vi "Begin.vi"() -> (0 "error out":errorcluster)   [LabVIEW 2012]
doc: "Called before other user functions, this VI is expected to open initial I/O refnums, load in file data, and do all program initialization. Notice that the <B>error out</B> terminal is simply used for data flow. Wiring it to other structures or subVIs ensures that this VI runs first."
uses:
  <vilib>/Rock Robotics/WPI/DriverStation/WPI_DriverStationRobotMode2.ctl
  <vilib>/Rock Robotics/WPI/Joystick/WPI_JoystickDeviceEnum.ctl
  <vilib>/Rock Robotics/SystemInterfaces/DIO/FPGA_DIOPWMChannel.ctl
  <vilib>/Rock Robotics/SystemInterfaces/DIO/FPGA_DIORelayChannel.ctl
  <vilib>/Rock Robotics/WPI/Relay/WPI_RelayDirection.ctl
  <vilib>/Rock Robotics/SystemInterfaces/DIO/FPGA_DIOChannel.ctl
  <vilib>/Rock Robotics/WPI/Encoder/WPI_EncoderType.ctl
  <vilib>/Rock Robotics/SystemInterfaces/AI/FPGA_AIGyroChannel.ctl
  <vilib>/Rock Robotics/WPI/Solenoid/WPI_SolenoidChannel.ctl
  <vilib>/Rock Robotics/SystemInterfaces/Typedef/FPGA_TypedefSolenoidModule.ctl
  Robot Global Data.vi
  <vilib>/Rock Robotics/WPI/RobotDrive/WPI_RobotDriveOpen4MotorWithTalon.vi
  <vilib>/Rock Robotics/WPI/Solenoid/WPI_SolenoidOpenSingle.vi
  <vilib>/Rock Robotics/WPI/Solenoid/Deprecated/WPI_SolenoidSetBool.vi
  <vilib>/Rock Robotics/WPI/Counter/WPI_CounterDigitalInputToDigitalSource.vi
  <vilib>/Rock Robotics/WPI/MotorControl/WPI_MotorControlOpen Jaguar.vi
  <vilib>/Rock Robotics/WPI/Compressor/WPI_CompressorGetSetRefNum.vi
  <vilib>/Rock Robotics/SystemInterfaces/Typedef/FPGA_TypedefDigitalModule.ctl
  <vilib>/Rock Robotics/WPI/MotorControl/WPI_MotorControlOpen Talon.vi
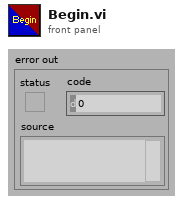
[diagram p1: front panel]
types:
  T1 = cluster{"Target Voltage":dbl, "Target Speed":dbl, "Angle Up?":bool}
  T2 = typedef "FPGA_DIOChannel.ctl" = enum8{"DIO 1", "DIO 2", "DIO 3", "DIO 4", "DIO 5", "DIO 6", "DIO 7", "DIO 8", "DIO 9", "DIO 10", "DIO 11", "DIO 12", "DIO 13", "DIO 14", "Invalid"}
  T3 = typedef "WPI_SolenoidChannel.ctl" = enum8{"Solenoid 1", "Solenoid 2", "Solenoid 3", "Solenoid 4", "Solenoid 5", "Solenoid 6", "Solenoid 7", "Solenoid 8", "Invalid"}
  T4 = typedef "FPGA_TypedefSolenoidModule.ctl" = enum16{"Solenoid Module 1", "Solenoid Module 2"}
  T5 = typedef "FPGA_AIGyroChannel.ctl" = enum8{"AI 1", "AI 2", "Invalid"}
  T6 = typedef "WPI_EncoderType.ctl" = enum16{"1x", "2x", "4x"}
  T7 = typedef "FPGA_DIORelayChannel.ctl" = enum8{"Relay 1", "Relay 2", "Relay 3", "Relay 4", "Relay 5", "Relay 6", "Relay 7", "Relay 8", "Invalid"}
  T8 = typedef "WPI_JoystickDeviceEnum.ctl" = enum16{"USB 1", "USB 2", "USB 3", "USB 4", "Kinect 1", "Kinect 2"}
  T9 = typedef "FPGA_DIOPWMChannel.ctl" = enum8{"PWM 1", "PWM 2", "PWM 3", "PWM 4", "PWM 5", "PWM 6", "PWM 7", "PWM 8", "PWM 9", "PWM 10", "Invalid"}
  T10 = typedef "WPI_RelayDirection.ctl" = enum16{"Both directions", "Forward only", "Reverse only"}
  T11 = typedef "WPI_DriverStationRobotMode2.ctl" = enum16{"Autonomous Disabled", "Autonomous Enabled", "Teleop Disabled", "Teleop Enabled", "Timeout", "Finish", "Test Disabled", "Test Enabled"}
  T12 = typedef "WPI_MotorControlDeviceRef.ctl" = cluster{"DeviceStatus":errorcluster, "Type":enum16{"PWM", "CAN"}, "PWM":cluster{"Digital Module":T13, "PWM Channel":T9, "DeadBand":T14}, "CAN":cluster{"Device Number":u8, "Control Mode":T15, "Semaphore":T16, "Max Vout":dbl}, "Invert":bool, "TransformRef":T17, "InvTransformRef":T17}
  T13 = typedef "FPGA_TypedefDigitalModule.ctl" = enum16{"Digital Module 1", "Digital Module 2"}
  T14 = typedef "WPI_PWMDeadband.ctl" = cluster{"Name":string, "maxPositivePwm":i32, "minPositivePwm":i32, "centerPwm":i32, "maxNegativePwm":i32, "minNegativePwm":i32, "angularRange":u16}
  T15 = typedef "WPI_CANJaguar_ControlMode.ctl" = enum8{"Percent VBus", "Current", "Speed", "Position", "Voltage"}
  T16 = typedef "Semaphore RefNum" = refnum<k1>
  T17 = typedef "WPI_PWMTransform_ConPane.ctl" = refnum<vi>
  T18 = typedef "WPI_DigitalInputDevRef.ctl" = cluster{"DevStatus":errorcluster, "DIO Channel":T2, "Digital Module":T13}
  T19 = typedef "WPI_ServoDeviceRef.ctl" = cluster{"DeviceStatus":errorcluster, "Digital Module":T13, "PWM Channel":T9, "DeadBand":T14}
  T20 = typedef "WPI_CompressorDevRef.ctl" = cluster{"DevStatus":errorcluster, "DigitalInputDevRef":T18, "RelayDevRef":T21}
  T21 = typedef "WPI_RelayDevRef.ctl" = cluster{"DevStatus":errorcluster, "Relay Channel":T7, "Digital Module":T13, "Relay Direction":T10}
  T22 = typedef "WPI_JoystickDevRef.ctl" = cluster{"Device":T8}
  T23 = typedef "WPI_SolenoidDevRef.ctl" = cluster{"DevStatus":errorcluster, "Solenoid Module":T4, "Forward Solenoid Channel":T3, "Reverse Solenoid Channel":T3}
  T24 = typedef "FPGA_CounterEncoderSourceConvertionLVSourceType.ctl" = cluster{"DevStatus":errorcluster, "AnalogTriggerMode?":bool, "DigitalMode":cluster{"Digital Module":T13, "DIO Channel":T25}, "AnalogTriggerMode":cluster{"AnalogTriggerIndex":T26, "OutputType":T27}}
  T25 = typedef "FPGA_DIODigitalSourceChannel.ctl" = enum8{"DIO 1", "DIO 2", "DIO 3", "DIO 4", "DIO 5", "DIO 6", "DIO 7", "DIO 8", "DIO 9", "DIO 10", "DIO 11", "DIO 12", "DIO 13", "DIO 14", "Disabled"}
  T26 = typedef "FPGA_AnalogTriggerIndex.ctl" = enum8{"Trig 0", "Trig 1", "Trig 2", "Trig 3", "Trig 4", "Trig 5", "Trig 6", "Trig 7", "Invalid"}
  T27 = typedef "FPGA_AnalogTriggerOutType.ctl" = enum16{"InWindow", "TriggerState", "Rising", "Falling"}
  T28 = typedef "WPI_GyroDevRef.ctl" = cluster{"DevStatus":errorcluster, "Analog Module":T29, "Analog Channel":T30, "Offset":dbl, "Gain (VoltsPerDegree/Second)":dbl}
  T29 = typedef "FPGA_TypedefAnalogModule.ctl" = enum16{"Analog Module 1", "Analog Module 2"}
  T30 = typedef "FPGA_AIChannel.ctl" = enum8{"AI 1", "AI 2", "AI 3", "AI 4", "AI 5", "AI 6", "AI 7", "AI 8", "Invalid"}
  T31 = typedef "WPI_RobotDriveDevRef.ctl" = cluster{"DevStatus":errorcluster, "Motors[]":T12[], "Square Inputs":bool, "Max Output":dbl, "Isochronous":bool}
  T32 = typedef "WPI_EncoderDevRef.ctl" = cluster{"DevStatus":errorcluster, "EncoderIndex":T33, "CounterIndex":T34, "DistancePerCount":dbl, "Decoding Type":T6}
  T33 = typedef "FPGA_EncoderIdx.ctl" = enum8{"Enc 0", "Enc 1", "Enc 2", "Enc 3", "Invalid"}
  T34 = typedef "FPGA_CounterCtrSystemIndex.ctl" = enum8{"Ctr 0", "Ctr 1", "Ctr 2", "Ctr 3", "Ctr 4", "Ctr 5", "Ctr 6", "Ctr 7", "Invalid"}
  T35 = cluster{"Target Voltage":dbl, "Target Speed":i32, "Angle Up?":bool}
  T36 = cluster{"Target Voltage":i32, "Target Speed":i32, "Angle Up?":bool}
  T37 = cluster{"Target Voltage":dbl, "Target Speed":dbl, "Angle Up?":bool}[]
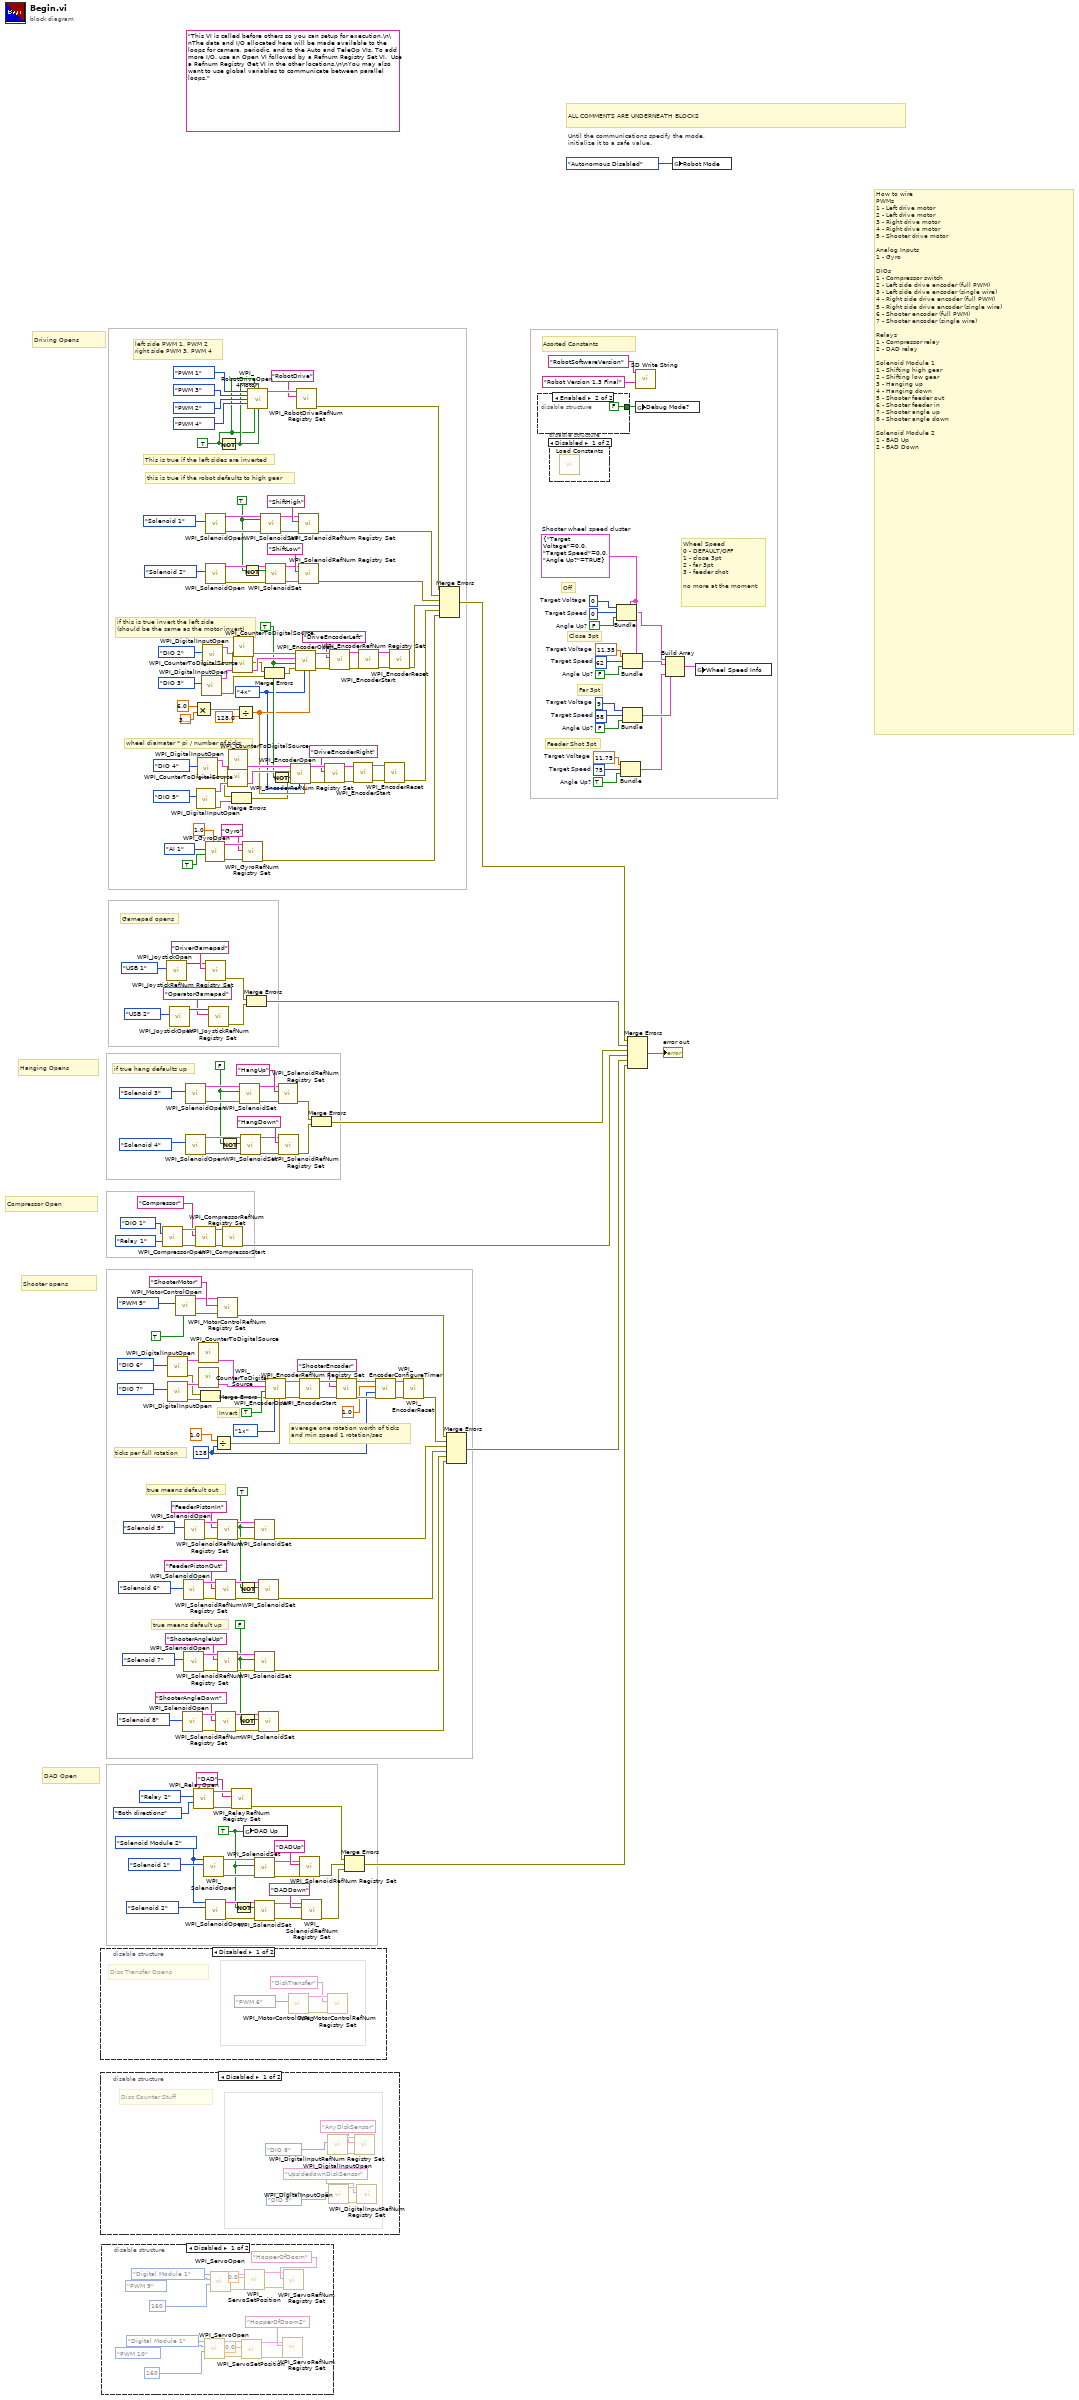
[diagram p0: block diagram]
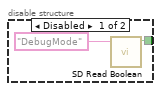
[diagram p2: hidden frame]
diagram:
  w5 = FALSE  # Angle Up?
  w4 = 0  # Target Speed
  w3 = 0  # Target Voltage
  w7 = u8 128 ("Number Samples to Average")
  w14 = TRUE  # Angle Up?
  w15 = 75  # Target Speed
  w16 = 11.75  # Target Voltage
  w19 = FALSE  # Angle Up?
  w18 = 58  # Target Speed
  w17 = 9  # Target Voltage
  w20 = FALSE  # Angle Up?
  w21 = 62  # Target Speed
  w22 = 11.35  # Target Voltage
  w2 = T1 {"Target Voltage"=0.0, "Target Speed"=0.0, "Angle Up?"=TRUE}  # Shooter wheel speed cluster
  w84 = FALSE
  w98 = TRUE
  w57 = TRUE
  w59 = FPGA_TypedefSolenoidModule."Solenoid Module 2" ("Solenoid Module (Module 1)")
  w60 = FALSE
  w62 = WPI_EncoderType."4x" ("Decoding Type")
  w64 = TRUE ("Invert Direction (False)")
  w82 = TRUE
  w80 = TRUE ("Rear Left Motor Inverted")
  (unwired) "This VI is called before others so you can setup for execution.\n\nThe data and I/O allocated here will be made available to the loops for camera, periodic, and to the Auto and TeleOp VIs. To add more I/O, use an Open VI followed by a Refnum Registry Set VI.  Use a Refnum Registry Get VI in the other locations.\n\nYou may also want to use global variables to communicate between parallel loops."
  # "Off"
  # "average one rotation worth of ticks\nand min speed 1 rotation/sec"
  # "Feeder Shot 3pt"
  # "Far 3pt"
  # "Close 3pt"
  # "How to wire\nPWMs\n1 - Left drive motor\n2 - Left drive motor\n3 - Right drive motor\n4 - Right drive motor\n5 - Shooter drive motor\n\nAnalog Inputs\n1 - Gyro\n\nDIOs\n1 - Compressor switch\n2 - Left side drive encoder (full PWM)\n3 - Left side drive encoder (single wire)\n4 - Right side drive encoder (full PWM)\n5 - Right side drive encoder (single wire)\n6 - Shooter encoder (full PWM)\n7 - Shooter encoder (single wire)\n\nRelays\n1 - Compressor relay\n2 - DAD relay\n\nSolenoid Module 1\n1 - Shifting high gear\n2 - Shifting low gear\n3 - Hanging up\n4 - Hanging down\n5 - Shooter feeder out\n6 - Shooter feeder in\n7 - Shooter angle up\n8 - Shooter angle down\n\nSolenoid Module 2\n1 - BAD Up\n2 - BAD Down"
  # "Asorted Constants"
  # "true means default up"
  # "true means default out"
  # "if true hang defaults up"
  # "Gamepad opens"
  # "wheel diamater * pi / number of ticks"
  # "if this is true invert the left side\n(should be the same as the motor invert)"
  # "this is true if the robot defaults to high gear"
  # "left side PWM 1, PWM 2\nright side PWM 3, PWM 4"
  # "This is true if the left sides are inverted"
  # "Compressor Open"
  # "Wheel Speed\n0 - DEFAULT/OFF\n1 - close 3pt\n2 - far 3pt\n3 - feeder shot\n\nno more at the moment"
  # "DAD Open"
  # "Hanging Opens"
  # "Driving Opens"
  # "Shooter opens"
  # "Invert"
  # "ticks per full rotation"
  # "ALL COMMENTS ARE UNDERNEATH BLOCKS"
  # "Until the communications specify the mode,\ninitialize it to a safe value."
  n1 = disable-structure shown="Disabled" {
    frame Disabled {
      # "Disc Transfer Opens"
      n2 = call-poly <vilib>:"WPI_MotorControlOpen.vi"("PWM Channel"=FPGA_DIOPWMChannel."PWM 6") -> ("error out"=w222:errorcluster, "MotorControlDeviceRef"=w223:T12)  [unwired: 9 in]
      n3 = call <vilib>:"WPI_MotorControlRefNum Registry Set.vi"("error in (no error)"=w222, "refnum name"="DiskTransfer", "MotorControlDevRef"=w223) -> ()  [unwired: 7 in, 2 out]
    }
    frame Enabled {
    }
  }
  n4 = disable-structure shown="Disabled" {
    frame Disabled {
      # "Disc Counter Stuff"
      n5 = call <vilib>:"WPI_DigitalInputOpen.vi"("DIO Channel"=FPGA_DIOChannel."DIO 8") -> ("error out"=w232:errorcluster, "DigitalInputDevRef"=w231:T18)  [unwired: 9 in]
      n6 = call <vilib>:"WPI_DigitalInputOpen.vi"("DIO Channel"=FPGA_DIOChannel."DIO 9") -> ("error out"=w230:errorcluster, "DigitalInputDevRef"=w229:T18)  [unwired: 9 in]
      n7 = call <vilib>:"WPI_DigitalInputRefNum Registry Set.vi"("error in (no error)"=w232, "refnum name"="AnyDiskSensor", "DigitalInputDevRef"=w231) -> ()  [unwired: 7 in, 2 out]
      n8 = call <vilib>:"WPI_DigitalInputRefNum Registry Set.vi"("error in (no error)"=w230, "refnum name"="UpsidedownDiskSensor", "DigitalInputDevRef"=w229) -> ()  [unwired: 7 in, 2 out]
    }
    frame Enabled {
    }
  }
  n9 = disable-structure shown="Disabled" {
    frame Disabled {
      n10 = call <vilib>:"WPI_ServoOpen.vi"("Angular Range"=160, "PWM Channel"=FPGA_DIOPWMChannel."PWM 10", "Digital Module (Module 1)"=FPGA_TypedefDigitalModule."Digital Module 1") -> ("error out"=w238:errorcluster, "ServoDeviceRef"=w237:T19)  [unwired: 7 in]
      n11 = call <vilib>:"WPI_ServoOpen.vi"("Angular Range"=160, "PWM Channel"=FPGA_DIOPWMChannel."PWM 9", "Digital Module (Module 1)"=FPGA_TypedefDigitalModule."Digital Module 1") -> ("error out"=w242:errorcluster, "ServoDeviceRef"=w241:T19)  [unwired: 7 in]
      n12 = call <vilib>:"WPI_ServoSetPosition.vi"("error in (no error)"=w238, "Position"=0.0, "ServoDeviceRef"=w237) -> ("error out"=w235:errorcluster, "ServoDeviceRef"=w236:T19)  [unwired: 7 in]
      n13 = call <vilib>:"WPI_ServoSetPosition.vi"("error in (no error)"=w242, "Position"=0.0, "ServoDeviceRef"=w241) -> ("error out"=w240:errorcluster, "ServoDeviceRef"=w239:T19)  [unwired: 7 in]
      n14 = call <vilib>:"WPI_ServoRefNum Registry Set.vi"("error in (no error)"=w235, "refnum name"="HopperOfDoom2", "ServoDeviceRef"=w236) -> ()  [unwired: 7 in, 2 out]
      n15 = call <vilib>:"WPI_ServoRefNum Registry Set.vi"("error in (no error)"=w240, "refnum name"="HopperOfDoom", "ServoDeviceRef"=w239) -> ()  [unwired: 7 in, 2 out]
    }
    frame Enabled {
    }
  }
  n16 = call <vilib>:"WPI_CompressorOpen.vi"("Pressure Switch DIO Channel"=FPGA_DIOChannel."DIO 1", "Relay Channel"=FPGA_DIORelayChannel."Relay 1") -> ("CompressorDevRef"=w164:T20, "error out"=w162:errorcluster)  [unwired: 12 in]
  n17 = call <vilib>:"WPI_JoystickOpen.vi"("JoystickDevice"=WPI_JoystickDeviceEnum."USB 1") -> ("JoystickDevRef"=w218:T22)  [unwired: 10 in]
  n18 = call <vilib>:"WPI_DigitalInputOpen.vi"("DIO Channel"=FPGA_DIOChannel."DIO 6") -> ("error out"=w180:errorcluster, "DigitalInputDevRef"=w193:T18)  [unwired: 9 in]
  n19 = call <vilib>:"WPI_DigitalInputOpen.vi"("DIO Channel"=FPGA_DIOChannel."DIO 7") -> ("error out"=w179:errorcluster, "DigitalInputDevRef"=w189:T18)  [unwired: 9 in]
  n20 = call <vilib>:"WPI_JoystickOpen.vi"("JoystickDevice"=WPI_JoystickDeviceEnum."USB 2") -> ("JoystickDevRef"=w166:T22)  [unwired: 10 in]
  n21 = call-poly <vilib>:"WPI_MotorControlOpen.vi"("Invert"=TRUE, "PWM Channel"=FPGA_DIOPWMChannel."PWM 5") -> ("error out"=w173:errorcluster, "MotorControlDeviceRef"=w174:T12)  [unwired: 8 in]
  n22 = call-poly <vilib>:"WPI_SolenoidOpen.vi"("Solenoid Channel"=WPI_SolenoidChannel."Solenoid 8") -> ("error out"=w94:errorcluster, "SolenoidDevRef"=w93:T23)  [unwired: 9 in]
  n23 = call-poly <vilib>:"WPI_SolenoidOpen.vi"("Solenoid Channel"=WPI_SolenoidChannel."Solenoid 6") -> ("error out"=w108:errorcluster, "SolenoidDevRef"=w107:T23)  [unwired: 9 in]
  n24 = call-poly <vilib>:"WPI_SolenoidOpen.vi"("Solenoid Channel"=WPI_SolenoidChannel."Solenoid 7") -> ("error out"=w89:errorcluster, "SolenoidDevRef"=w90:T23)  [unwired: 9 in]
  n25 = call-poly <vilib>:"WPI_SolenoidOpen.vi"("Solenoid Channel"=WPI_SolenoidChannel."Solenoid 5") -> ("error out"=w103:errorcluster, "SolenoidDevRef"=w104:T23)  [unwired: 9 in]
  n26 = call-poly <vilib>:"WPI_SolenoidOpen.vi"("Solenoid Channel"=WPI_SolenoidChannel."Solenoid 4") -> ("error out"=w130:errorcluster, "SolenoidDevRef"=w131:T23)  [unwired: 9 in]
  n27 = call-poly <vilib>:"WPI_SolenoidOpen.vi"("Solenoid Channel"=WPI_SolenoidChannel."Solenoid 3") -> ("error out"=w133:errorcluster, "SolenoidDevRef"=w132:T23)  [unwired: 9 in]
  n28 = Multiply(x=6.0, y=3.141592653589793) -> (x*y=w151:dbl)
  n29 = call <vilib>:"WPI_RelayOpen.vi"("Relay Direction"=WPI_RelayDirection."Both directions", "Relay Channel"=FPGA_DIORelayChannel."Relay 2") -> ("error out"=w196:errorcluster, "RelayDevRef"=w195:T21)  [unwired: 8 in]
  n30 = call <vilib>:"WPI_CompressorRefNum Registry Set.vi"("error in (no error)"=w162, "refnum name"="Compressor", "CompressorDevRef"=w164) -> ("error out"=w112:errorcluster, "CompressorDevRef"=w113:T20)  [unwired: 7 in]
  n31 = call <vilib>:"WPI_DigitalInputOpen.vi"("DIO Channel"=FPGA_DIOChannel."DIO 5") -> ("error out"=w50:errorcluster, "DigitalInputDevRef"=w72:T18)  [unwired: 9 in]
  n32 = call <vilib>:"WPI_DigitalInputOpen.vi"("DIO Channel"=FPGA_DIOChannel."DIO 4") -> ("error out"=w49:errorcluster, "DigitalInputDevRef"=w71:T18)  [unwired: 9 in]
  n33 = call-poly <vilib>:"WPI_CounterToDigitalSource.vi"("DigitalInputDevRef"=w193) -> ("Digital Source"=w192:T24)  [unwired: 6 in]
  n34 = call-poly <vilib>:"WPI_CounterToDigitalSource.vi"("DigitalInputDevRef"=w189) -> ("Digital Source"=w186:T24)  [unwired: 6 in]
  n35 = Merge Errors(w180, w179) -> (w181:errorcluster)
  n36 = call <vilib>:"WPI_DigitalInputOpen.vi"("DIO Channel"=FPGA_DIOChannel."DIO 3") -> ("error out"=w45:errorcluster, "DigitalInputDevRef"=w154:T18)  [unwired: 9 in]
  n37 = call <vilib>:"WPI_DigitalInputOpen.vi"("DIO Channel"=FPGA_DIOChannel."DIO 2") -> ("error out"=w46:errorcluster, "DigitalInputDevRef"=w155:T18)  [unwired: 9 in]
  n38 = call-poly <vilib>:"WPI_SolenoidOpen.vi"("Solenoid Channel"=WPI_SolenoidChannel."Solenoid 1", "Solenoid Module (Module 1)"=w59) -> ("error out"=w117:errorcluster, "SolenoidDevRef"=w121:T23)  [unwired: 8 in]
  n39 = call <vilib>:"WPI_GyroOpen.vi"("Calibration Time (s)"=1.0, "Calibrate On Open"=TRUE, "Analog Channel"=FPGA_AIGyroChannel."AI 1") -> ("error out"=w143:errorcluster, "GyroDevRef"=w142:T28)  [unwired: 6 in, 1 out]
  n40 = call-poly <vilib>:"WPI_SolenoidOpen.vi"("Solenoid Channel"=WPI_SolenoidChannel."Solenoid 1") -> ("error out"=w203:errorcluster, "SolenoidDevRef"=w206:T23)  [unwired: 9 in]
  n41 = call-poly <vilib>:"WPI_SolenoidOpen.vi"("Solenoid Channel"=WPI_SolenoidChannel."Solenoid 2") -> ("error out"=w200:errorcluster, "SolenoidDevRef"=w202:T23)  [unwired: 9 in]
  n42 = call <vilib>:"WPI_JoystickRefNum Registry Set.vi"("refnum name"="DriverGamepad", "JoystickDevRef"=w218) -> ("error out"=w42:errorcluster)  [unwired: 8 in, 1 out]
  n43 = call-poly <vilib>:"WPI_SolenoidOpen.vi"("Solenoid Channel"=WPI_SolenoidChannel."Solenoid 2", "Solenoid Module (Module 1)"=w59) -> ("error out"=w114:errorcluster, "SolenoidDevRef"=w119:T23)  [unwired: 8 in]
  n44 = call <vilib>:"WPI_JoystickRefNum Registry Set.vi"("refnum name"="OperatorGamepad", "JoystickDevRef"=w166) -> ("error out"=w41:errorcluster)  [unwired: 8 in, 1 out]
  n45 = Divide(x=1.0, y=w7) -> (x/y=w8:dbl)
  n46 = call <vilib>:"WPI_SolenoidRefNum Registry Set.vi"("error in (no error)"=w108, "refnum name"="FeederPistonOut", "SolenoidDevRef"=w107) -> ("error out"=w110:errorcluster, "SolenoidDevRef"=w109:T23)  [unwired: 7 in]
  n47 = call <vilib>:"WPI_SolenoidRefNum Registry Set.vi"("error in (no error)"=w94, "refnum name"="ShooterAngleDown", "SolenoidDevRef"=w93) -> ("error out"=w96:errorcluster, "SolenoidDevRef"=w95:T23)  [unwired: 7 in]
  n48 = call <vilib>:"WPI_MotorControlRefNum Registry Set.vi"("error in (no error)"=w173, "refnum name"="ShooterMotor", "MotorControlDevRef"=w174) -> ("error out"=w38:errorcluster)  [unwired: 7 in, 1 out]
  n49 = call <vilib>:"WPI_SolenoidRefNum Registry Set.vi"("error in (no error)"=w103, "refnum name"="FeederPistonIn", "SolenoidDevRef"=w104) -> ("error out"=w101:errorcluster, "SolenoidDevRef"=w102:T23)  [unwired: 7 in]
  n50 = call <vilib>:"WPI_SolenoidRefNum Registry Set.vi"("error in (no error)"=w89, "refnum name"="ShooterAngleUp", "SolenoidDevRef"=w90) -> ("error out"=w87:errorcluster, "SolenoidDevRef"=w88:T23)  [unwired: 7 in]
  n51 = Not(x=w80) -> (.not. x?=w81:bool)
  n52 = Not(x=w60) -> (.not. x?=w61:bool)
  n53 = call <vilib>:"WPI_CompressorStart.vi"("error in (no error)"=w112, "CompressorDevRef"=w113) -> ("error out"=w26:errorcluster)  [unwired: 8 in, 1 out]
  n54 = call-poly <vilib>:"WPI_CounterToDigitalSource.vi"("DigitalInputDevRef"=w72) -> ("Digital Source"=w69:T24)  [unwired: 6 in]
  n55 = call-poly <vilib>:"WPI_CounterToDigitalSource.vi"("DigitalInputDevRef"=w71) -> ("Digital Source"=w67:T24)  [unwired: 6 in]
  n56 = call <vilib>:"WPI_RelayRefNum Registry Set.vi"("error in (no error)"=w196, "refnum name"="DAD", "RelayDevRef"=w195) -> ("error out"=w32:errorcluster)  [unwired: 7 in, 1 out]
  n57 = Merge Errors(w49, w50) -> (w48:errorcluster)
  n58 = call-poly <vilib>:"WPI_CounterToDigitalSource.vi"("DigitalInputDevRef"=w154) -> ("Digital Source"=w157:T24)  [unwired: 6 in]
  n59 = call-poly <vilib>:"WPI_CounterToDigitalSource.vi"("DigitalInputDevRef"=w155) -> ("Digital Source"=w159:T24)  [unwired: 6 in]
  n60 = Not(x=w57) -> (.not. x?=w58:bool)
  n61 = Divide(x=w151, y=128.0 ("x")) -> (x/y=w63:dbl)
  n62 = Not(x=w84) -> (.not. x?=w97:bool)
  n63 = Not(x=w98) -> (.not. x?=w111:bool)
  n64 = call-poly <vilib>:"WPI_SolenoidSet.vi"("error in (no error)"=w133, "Value"=w60, "SolenoidDevRef"=w132) -> ("error out"=w126:errorcluster, "SolenoidDevRef"=w129:T23)  [unwired: 7 in]
  n65 = call-poly <vilib>:"WPI_SolenoidSet.vi"("error in (no error)"=w130, "Value"=w61, "SolenoidDevRef"=w131) -> ("error out"=w127:errorcluster, "SolenoidDevRef"=w128:T23)  [unwired: 7 in]
  n66 = Not(x=w82) -> (.not. x?=w83:bool)
  n67 = call <vilib>:"WPI_GyroRefNum Registry Set.vi"("error in (no error)"=w143, "refnum name"="Gyro", "GyroDevRef"=w142) -> ("error out"=w43:errorcluster)  [unwired: 7 in, 1 out]
  n68 = global write "Robot Global Data.vi" "DAD Up"(w57) -> ()
  n69 = Merge Errors(w42, w41) -> (w28:errorcluster)
  n70 = call-poly <vilib>:"WPI_RobotDriveOpen4Motor.vi"("Rear Left Motor"=FPGA_DIOPWMChannel."PWM 1", "Rear Left Motor Inverted"=w80, "Rear Right Motor Inverted"=w81, "Rear Right Motor"=FPGA_DIOPWMChannel."PWM 3", "Front Left Motor"=FPGA_DIOPWMChannel."PWM 2", "Front Right Motor"=FPGA_DIOPWMChannel."PWM 4" ("Front Left Motor"), "Front Left Motor Inverted"=w80, "Front Right Motor Inverted"=w81) -> ("RobotDriveDevRef"=w212:T31)  [unwired: 6 in, 1 out]
  n71 = call-poly <vilib>:"WPI_SolenoidSet.vi"("error in (no error)"=w87, "Value"=w84, "SolenoidDevRef"=w88) -> ("error out"=w34:errorcluster)  [unwired: 7 in, 1 out]
  n72 = call-poly <vilib>:"WPI_SolenoidSet.vi"("error in (no error)"=w117, "Value"=w57, "SolenoidDevRef"=w121) -> ("error out"=w116:errorcluster, "SolenoidDevRef"=w120:T23)  [unwired: 7 in]
  n73 = call-poly <vilib>:"WPI_SolenoidSet.vi"("error in (no error)"=w114, "Value"=w58, "SolenoidDevRef"=w119) -> ("error out"=w115:errorcluster, "SolenoidDevRef"=w118:T23)  [unwired: 7 in]
  n74 = call-poly <vilib>:"WPI_SolenoidSet.vi"("error in (no error)"=w101, "Value"=w98, "SolenoidDevRef"=w102) -> ("error out"=w36:errorcluster)  [unwired: 7 in, 1 out]
  n75 = call-poly <vilib>:"WPI_SolenoidSet.vi"("error in (no error)"=w96, "Value"=w97, "SolenoidDevRef"=w95) -> ("error out"=w33:errorcluster)  [unwired: 7 in, 1 out]
  n76 = call-poly <vilib>:"WPI_SolenoidSet.vi"("error in (no error)"=w110, "Value"=w111, "SolenoidDevRef"=w109) -> ("error out"=w35:errorcluster)  [unwired: 7 in, 1 out]
  n77 = call-poly <vilib>:"WPI_SolenoidSet.vi"("error in (no error)"=w203, "Value"=w82, "SolenoidDevRef"=w206) -> ("error out"=w204:errorcluster, "SolenoidDevRef"=w205:T23)  [unwired: 7 in]
  n78 = Merge Errors(w46, w45) -> (w47:errorcluster)
  n79 = call-poly <vilib>:"WPI_SolenoidSet.vi"("error in (no error)"=w200, "Value"=w83, "SolenoidDevRef"=w202) -> ("error out"=w199:errorcluster, "SolenoidDevRef"=w201:T23)  [unwired: 7 in]
  n80 = call <vilib>:"WPI_EncoderOpen.vi"("DistancePerCount"=w8, "Decoding Type"=WPI_EncoderType."1x", "error in (no error)"=w181, "Invert Direction (False)"=TRUE, "BSource"=w186, "ASource"=w192) -> ("error out"=w182:errorcluster, "EncoderDevRef"=w183:T32)  [unwired: 4 in]
  n81 = Not(x=w64) -> (.not. x?=w65:bool)
  n82 = call <vilib>:"WPI_SolenoidRefNum Registry Set.vi"("error in (no error)"=w126, "refnum name"="HangUp", "SolenoidDevRef"=w129) -> ("error out"=w40:errorcluster)  [unwired: 7 in, 1 out]
  n83 = call <vilib>:"WPI_SolenoidRefNum Registry Set.vi"("error in (no error)"=w127, "refnum name"="HangDown", "SolenoidDevRef"=w128) -> ("error out"=w39:errorcluster)  [unwired: 7 in, 1 out]
  n84 = call <vilib>:"WPI_EncoderOpen.vi"("DistancePerCount"=w63, "Decoding Type"=w62, "error in (no error)"=w48, "Invert Direction (False)"=w65, "BSource"=w69, "ASource"=w67) -> ("error out"=w73:errorcluster, "EncoderDevRef"=w74:T32)  [unwired: 4 in]
  n85 = call <vilib>:"WPI_EncoderOpen.vi"("DistancePerCount"=w63, "Decoding Type"=w62, "error in (no error)"=w47, "Invert Direction (False)"=w64, "BSource"=w157, "ASource"=w159) -> ("error out"=w150:errorcluster, "EncoderDevRef"=w149:T32)  [unwired: 4 in]
  n86 = call <vilib>:"WPI_RobotDriveRefNum Registry Set.vi"("refnum name"="RobotDrive", "RobotDriveDevRef"=w212) -> ("error out"=w54:errorcluster)  [unwired: 8 in, 1 out]
  n87 = call <vilib>:"WPI_SolenoidRefNum Registry Set.vi"("error in (no error)"=w204, "refnum name"="ShiftHigh", "SolenoidDevRef"=w205) -> ("error out"=w53:errorcluster)  [unwired: 7 in, 1 out]
  n88 = call <vilib>:"WPI_SolenoidRefNum Registry Set.vi"("error in (no error)"=w199, "refnum name"="ShiftLow", "SolenoidDevRef"=w201) -> ("error out"=w52:errorcluster)  [unwired: 7 in, 1 out]
  n89 = call <vilib>:"WPI_EncoderStart.vi"("error in (no error)"=w182, "EncoderDevRef"=w183) -> ("error out"=w178:errorcluster, "EncoderDevRef"=w184:T32)  [unwired: 8 in]
  n90 = call <vilib>:"WPI_SolenoidRefNum Registry Set.vi"("error in (no error)"=w116, "refnum name"="DADUp", "SolenoidDevRef"=w120) -> ("error out"=w31:errorcluster)  [unwired: 7 in, 1 out]
  n91 = call <vilib>:"WPI_SolenoidRefNum Registry Set.vi"("error in (no error)"=w115, "refnum name"="DADDown", "SolenoidDevRef"=w118) -> ("error out"=w30:errorcluster)  [unwired: 7 in, 1 out]
  n92 = Merge Errors(w40, w39) -> (w27:errorcluster)
  n93 = call <vilib>:"WPI_EncoderRefNum Registry Set.vi"("error in (no error)"=w73, "refnum name"="DriveEncoderRight", "EncoderDevRef"=w74) -> ("error out"=w75:errorcluster, "EncoderDevRef"=w76:T32)  [unwired: 7 in]
  n94 = call <vilib>:"WPI_EncoderRefNum Registry Set.vi"("error in (no error)"=w150, "refnum name"="DriveEncoderLeft", "EncoderDevRef"=w149) -> ("error out"=w148:errorcluster, "EncoderDevRef"=w147:T32)  [unwired: 7 in]
  n95 = call <vilib>:"WPI_EncoderRefNum Registry Set.vi"("error in (no error)"=w178, "refnum name"="ShooterEncoder", "EncoderDevRef"=w184) -> ("error out"=w169:errorcluster, "EncoderDevRef"=w170:T32)  [unwired: 7 in]
  n96 = Merge Errors(w32, w31, w30) -> (w24:errorcluster)
  n97 = call <vilib>:"WPI_EncoderStart.vi"("error in (no error)"=w75, "EncoderDevRef"=w76) -> ("error out"=w77:errorcluster, "EncoderDevRef"=w78:T32)  [unwired: 8 in]
  n98 = call <vilib>:"WPI_EncoderStart.vi"("error in (no error)"=w148, "EncoderDevRef"=w147) -> ("error out"=w146:errorcluster, "EncoderDevRef"=w145:T32)  [unwired: 8 in]
  n99 = call <vilib>:"WPI_EncoderConfigureTimer.vi"("error in (no error)"=w169, "Number Samples to Average"=w7, "Minimum Rate"=1.0, "EncoderDevRef"=w170) -> ("error out"=w172:errorcluster, "EncoderDevRef"=w171:T32)  [unwired: 6 in]
  n100 = call <vilib>:"WPI_EncoderReset.vi"("error in (no error)"=w77, "EncoderDevRef"=w78) -> ("error out"=w44:errorcluster)  [unwired: 8 in, 1 out]
  n101 = call <vilib>:"WPI_EncoderReset.vi"("error in (no error)"=w146, "EncoderDevRef"=w145) -> ("error out"=w51:errorcluster)  [unwired: 8 in, 1 out]
  n102 = call <vilib>:"WPI_EncoderReset.vi"("error in (no error)"=w172, "EncoderDevRef"=w171) -> ("error out"=w37:errorcluster)  [unwired: 8 in, 1 out]
  n103 = Merge Errors(w54, w53, w52, w51, w44, w43) -> (w29:errorcluster)
  n104 = Merge Errors(w38, w37, w36, w35, w34, w33) -> (w25:errorcluster)
  n105 = disable-structure shown="Enabled" {
    disable-tunnel: [w251 FALSE ("Debug Mode?")] -> w9
    frame Disabled {
      n106 = call <vilib>:"SD Read Boolean.vi"("Name"="DebugMode") -> ("Boolean"=w251:bool)  [unwired: 8 in, 2 out]
    }
    frame Enabled {
    }
  }
  n107 = disable-structure shown="Disabled" {
    frame Disabled {
      n108 = call "Load Constants.vi"() -> ()  [unwired: 12 in]
    }
    frame Enabled {
    }
  }
  n109 = Bundle(cluster=w2, "Target Voltage"=w3, "Target Speed"=w4, "Angle Up?"=w5) -> (w1:T1)
  n110 = Bundle("Target Voltage"=w16, "Target Speed"=w15, "Angle Up?"=w14) -> (w11:T35)  [unwired: 1 in]
  n111 = Bundle(cluster=w2, "Target Voltage"=w22, "Target Speed"=w21, "Angle Up?"=w20) -> (w13:T1)
  n112 = Bundle("Target Voltage"=w17, "Target Speed"=w18, "Angle Up?"=w19) -> (w12:T36)  [unwired: 1 in]
  n113 = Merge Errors(w29, w28, w27, w26, w25, w24) -> (→"error out":errorcluster)
  n114 = call <vilib>:"SD Write String.vi"("String"="Robot Version 1.3 Final", "Name"="RobotSoftwareVersion") -> ()  [unwired: 8 in, 2 out]
  n115 = global write "Robot Global Data.vi" "Debug Mode?"(w9) -> ()
  n116 = Build Array(w1, w13, w12, w11) -> (w10:T37)
  n117 = global write "Robot Global Data.vi" "Robot Mode"(WPI_DriverStationRobotMode2."Autonomous Disabled" ("Robot Mode")) -> ()
  n118 = global write "Robot Global Data.vi" "Wheel Speed Info"(w10) -> ()
